vi "Test Init and Close.vi"(8 "error in (no error)":errorcluster) -> (0 "error out":errorcluster)   [LabVIEW 2016, in "UT_UserEventHandler.lvlib"]
doc: "Test the initializatuin and closing a UserEventHandler object."
uses:
  UT_UserEventHandler.lvlib
  Source/HSE-Logger/LogLevel.ctl
  <vilib>/addons/_JKI Toolkits/Caraya/classes/Assert/Assert False.vi
  <vilib>/addons/_JKI Toolkits/Caraya/classes/Assert/Assert Equal Value and Type_Variant.vi
  <vilib>/addons/_JKI Toolkits/Caraya/classes/Assert/Assert True.vi
  Source/HSE-Logger/Handler/UserEventHandler/UserEventHandler.lvclass
  <vilib>/addons/_JKI Toolkits/Caraya/classes/Test/Test.lvclass
  Source/HSE-Logger/hse-logger.lvlib
  <vilib>/addons/_JKI Toolkits/Caraya/classes/Assert/Assert.lvclass
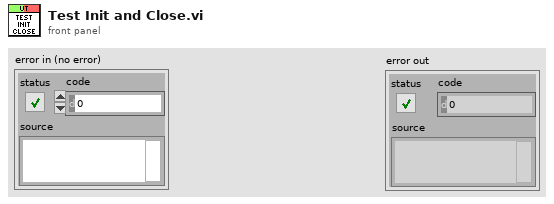
[diagram p1: front panel]
types:
  T1 = typedef "hse-logger.lvlib/LogLevel.ctl" = enum16{"DEBUG", "INFO", "WARNING", "ERROR", "CRITICAL"}
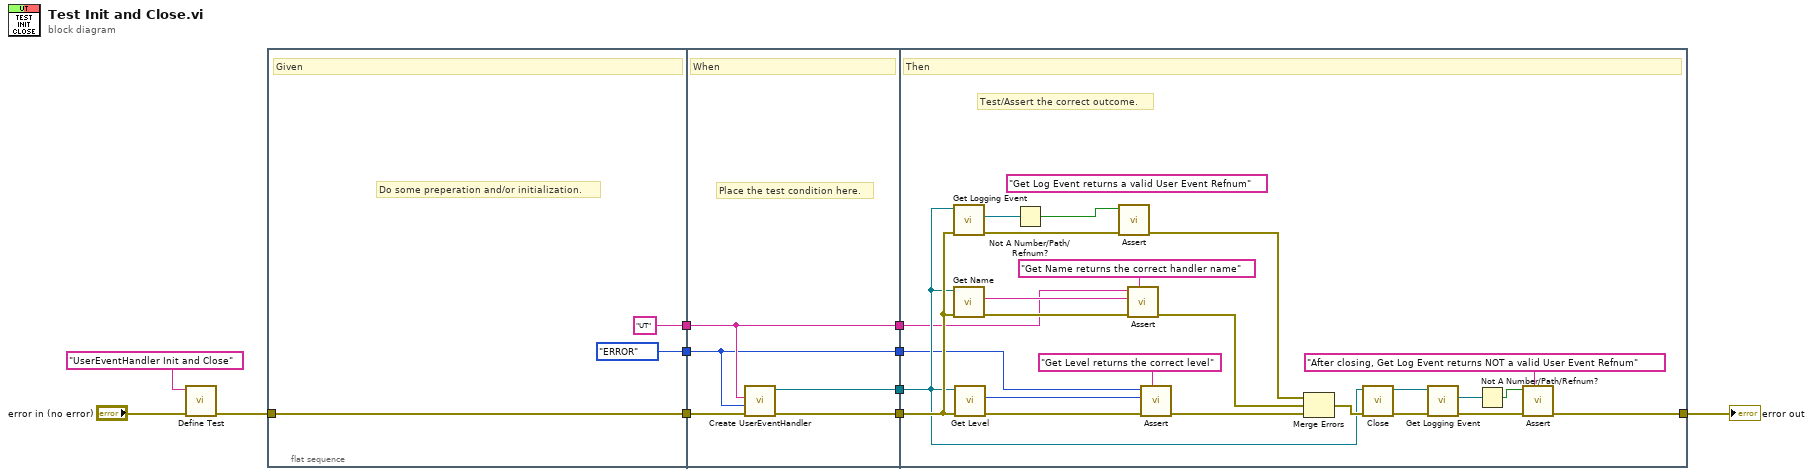
[diagram p0: block diagram]
diagram:
  n1 = call <vilib>:"Define Test.vi"("error in (no error)"="error in (no error)", "Label (VI Title)"="UserEventHandler Init and Close") -> ("error out"=w8:errorcluster)  [unwired: 8 in, 1 out]
  n2 = flat-sequence {
    tunnel: w8 -> [w14]
    tunnel: [w14] -> w11
    tunnel: ["UT" ("Name")] -> w5
    tunnel: [LogLevel."ERROR" ("Level")] -> w4
    tunnel: w11 -> [w19]
    tunnel: [w18] -> w6
    tunnel: w5 -> [w16]
    tunnel: w4 -> [w15]
    tunnel: [w17] -> w3
    tunnel: [w15] -> w2
    tunnel: [w16] -> w1
    tunnel: [w22] -> w10
    tunnel: w6 -> [w43]
    tunnel: w3 -> [w41]
    tunnel: w2 -> [w26]
    tunnel: w1 -> [w30]
    frame #0 {
      # "Do some preperation and/or initialization."
      # "Given"
    }
    frame #1 {
      # "Place the test condition here."
      # "When"
      n3 = call "Create UserEventHandler.vi"("error in"=w19, "Level"=w15, "Name"=w16) -> ("error out"=w18:errorcluster, "UserEventHandler out"=w17:refnum<class "UserEventHandler.lvclass">)  [unwired: 7 in]
    }
    frame #2 {
      (unwired) "Get Log Event returns a valid User Event Refnum" ("Label")
      # "Test/Assert the correct outcome."
      # "Then"
      n4 = call-dynamic "Get Logging Event.vi"("error in"=w43, "UserEventHandler in"=w41) -> ("error out"=w36:errorcluster, "Logging Event"=w40:refnum<user-event>)  [unwired: 7 in, 1 out]
      n5 = call-dynamic "Get Name.vi"("error in"=w43, "Handler in"=w41) -> ("error out"=w33:errorcluster, "Name"=w31:string)  [unwired: 7 in, 1 out]
      n6 = call-dynamic "Get Level.vi"("error in"=w43, "Handler in"=w41) -> ("error out"=w28:errorcluster, "Level"=w25:T1)  [unwired: 7 in, 1 out]
      n7 = Not A Number/Path/Refnum?(number/path/refnum=w40) -> (NaN/Path/Refnum?=w35:bool)
      n8 = call-poly <vilib>:"Assert.vi"("error in (no error)"=w36, "False?"=w35) -> ("error out"=w34:errorcluster)  [unwired: 8 in, 1 out]
      n9 = call-poly <vilib>:"Assert.vi"("Label"="Get Name returns the correct handler name", "error in (no error)"=w33, "Y"=w31, "X"=w30) -> ("error out"=w32:errorcluster)  [unwired: 6 in, 1 out]
      n10 = call-poly <vilib>:"Assert.vi"("Label"="Get Level returns the correct level", "error in (no error)"=w28, "Y"=w25, "X"=w26) -> ("error out"=w27:errorcluster)  [unwired: 6 in, 1 out]
      n11 = Merge Errors(w34, w32, w27) -> (w42:errorcluster)
      n12 = call-dynamic "Close.vi"("error in"=w42, "UserEventHandler in"=w41) -> ("error out"=w38:errorcluster, "UserEventHandler out"=w39:refnum<class "UserEventHandler.lvclass">)  [unwired: 8 in]
      n13 = call-dynamic "Get Logging Event.vi"("error in"=w38, "UserEventHandler in"=w39) -> ("error out"=w23:errorcluster, "Logging Event"=w37:refnum<user-event>)  [unwired: 7 in, 1 out]
      n14 = Not A Number/Path/Refnum?(number/path/refnum=w37) -> (NaN/Path/Refnum?=w20:bool)
      n15 = call-poly <vilib>:"Assert.vi"("Label"="After closing, Get Log Event returns NOT a valid User Event Refnum", "error in (no error)"=w23, "True?"=w20) -> ("error out"=w22:errorcluster)  [unwired: 7 in, 1 out]
    }
  }
  "error out" <- w10
